vi "Radix 2 Real.vi"(1 "X":dbl[](array[numeric]) format="%0.2f") -> (0 "Y":dbl[](array[numeric]) format="%0.2f")   [LabVIEW 2017, in "NI_Gmath.lvlib"]
uses:
  NI_Gmath.lvlib
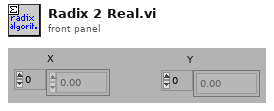
[diagram p1: front panel]
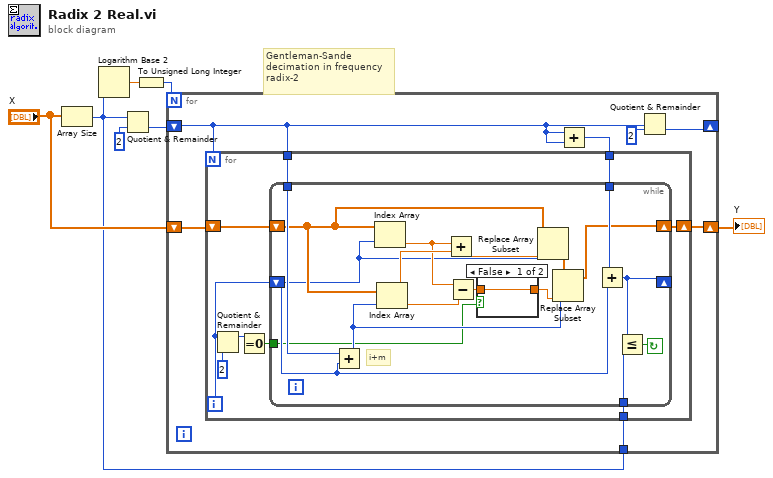
[diagram p0: block diagram]
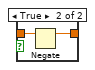
[diagram p2: hidden frame]
diagram:
  # "Gentleman-Sande\ndecimation in frequency\nradix-2"
  n1 = Array Size(array="X") -> (size(s)=w5:i32)
  n2 = Logarithm Base 2(1:w5) -> (0:w4:dbl)
  n3 = Quotient & Remainder(x=w5, y=2) -> (floor(x/y)=w2:i32)  [unwired: 1 out]
  n4 = To Unsigned Long Integer(number=w4) -> (unsigned 32bit integer=w1:u32)
  n5 = for {
    N: w1 -> [_]
    shift-right: [w11] -> w6
    shift-left: "X" -> [w12]
    shift-right: [w13] -> _
    shift-left: w2 -> [w8]
    tunnel: w5 -> [w9]
    n6 = Add(x=w8, y=w8) -> (x+y=w10:i32)
    n7 = for {
      N: w8 -> [_]
      shift-right: [w22] -> w11
      shift-left: w12 -> [w23]
      tunnel: w10 -> [w21]
      tunnel: w9 -> [w20]
      tunnel: w8 -> [w19]
      i -> [w18]
      n8 = Quotient & Remainder(x=w18, y=2) -> (x-y*floor(x/y)=w16:i32)  [unwired: 1 out]
      n9 = Equal To 0?(x=w16) -> (x = 0?=w15:bool)
      n10 = while {
        tunnel: w15 -> [w26]
        tunnel: w19 -> [w36]
        tunnel: w20 -> [w38]
        tunnel: w21 -> [w39]
        shift-left: w18 -> [w28]
        shift-right: [w27] -> _
        shift-left: w23 -> [w31]
        shift-right: [w29] -> w22
        stop <- w37 continue-if-true
        # "i+m"
        # "i"
        n11 = Add(x=w36, y=w28) -> (x+y=w33:i32)
        n12 = Index Array(array=w31, index=w28) -> (element=w34:dbl)
        n13 = Index Array(array=w31, index=w33) -> (element=w35:dbl)
        n14 = Add(x=w34, y=w35) -> (x+y=w32:dbl)
        n15 = Subtract(x=w34, y=w35) -> (x-y=w25:dbl)
        n16 = case shown="False" w26 {
          tunnel: [w40 w41] -> w24
          tunnel: w25 -> [w40 w42]
          frame False {
          }
          frame True {
            n17 = Negate(x=w42) -> (-x=w41:dbl)
          }
        }
        n18 = Replace Array Subset(array=w31, new element=w32, index=w28) -> (w30:dbl[])
        n19 = Replace Array Subset(array=w30, new element=w24, index=w33) -> (w29:dbl[])
        n20 = Add(x=w39, y=w28) -> (x+y=w27:i32)
        n21 = Less Or Equal?(x=w27, y=w38) -> (x <= y?=w37:bool)
      }
    }
    n22 = Quotient & Remainder(x=w8, y=2) -> (floor(x/y)=w13:i32)  [unwired: 1 out]
  }
  "Y" <- w6
